vi "one_by_one.vi"(8 "error in (no error)":errorcluster caption="エラー入力（エラーなし）", 9 "入力文字":string, 10 "待機 (200ms)":u16=200, 11 "VISAリソース名":refnum<visa-resource-name>) -> (0 "error out":errorcluster caption="エラー出力", 3 "VISAリソース名出力":refnum<visa-resource-name>)   [LabVIEW 2017]
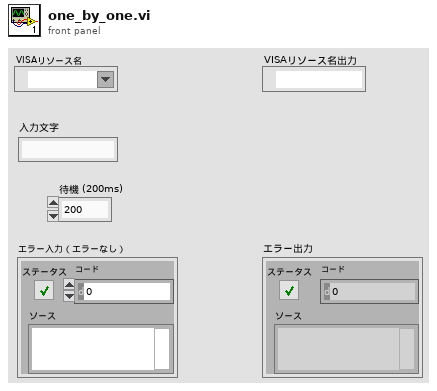
[diagram p1: front panel]
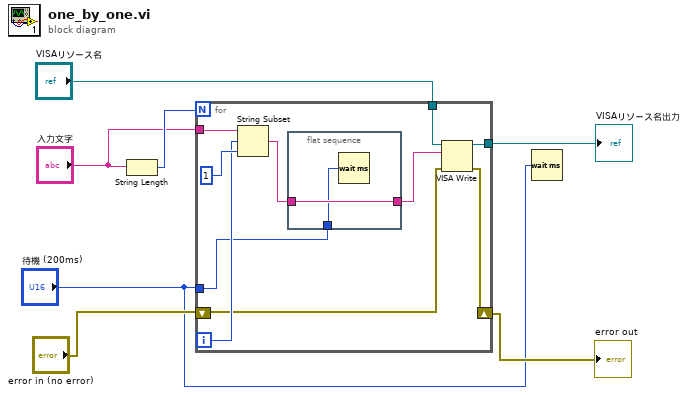
[diagram p0: block diagram]
diagram:
  n1 = String Length(string="入力文字") -> (length=w6:i32)
  n2 = for {
    N: w6 -> [_]
    tunnel: "入力文字" -> [w17]
    tunnel: [w13] -> w7
    tunnel: "VISAリソース名" -> [w12]
    tunnel: "待機 (200ms)" -> [w10]
    shift-right: [w8] -> w2
    shift-left: "error in (no error)" -> [w9]
    i -> [w11]
    n3 = String Subset(string=w17, offset (0)=w11, length (rest)=1) -> (substring=w15:string)
    n4 = flat-sequence {
      tunnel: w15 -> [w19]
      tunnel: [w19] -> w14
      tunnel: w10 -> [w18]
      frame #0 {
        n5 = Wait (ms)(milliseconds to wait=w18) -> ()  [unwired: 1 out]
      }
    }
    n6 = VISA Write(VISA resource name=w12, write buffer=w14, error in (no error)=w9) -> (VISA resource name out=w13:refnum<visa-resource-name>, error out=w8:errorcluster)  [unwired: 1 out]
  }
  "VISAリソース名出力" <- w7
  "error out" <- w2
  n7 = Wait (ms)(milliseconds to wait="待機 (200ms)") -> ()  [unwired: 1 out]
